vi "mupExpr Demo5.vi"() -> ()   [LabVIEW 2015]
uses:
  mupExpr/mupExpr.lvclass/mupExpr.ctl
  mupExpr/Set_SglVar_BulkMode_Value.vi
  mupExpr/Eval_BulkMode.vi
  mupExpr/Read Bulk Size.vi
  mupExpr/Read Expression.vi
  mupExpr/Read Singe Var Name.vi
  mupExpr/Read Variable_Names.vi
  mupLib/mupSetVarValue_Array.vi
  mupLib/mupEvalBulk.vi
  mupLib/mupCheckError.vi
  mupLib/mupLibPath.vi
  <vilib>/Utility/error.llb/Error Cluster From Error Code.vi
  mupExpr/mupExpr.lvclass
panel:
  in  "varValue":dbl[](array[numeric])=[0.0, 1.0, 2.0, 3.0, 4.0, 5.0]
  out "Result":dbl[](array[numeric]) format="%#_13g"
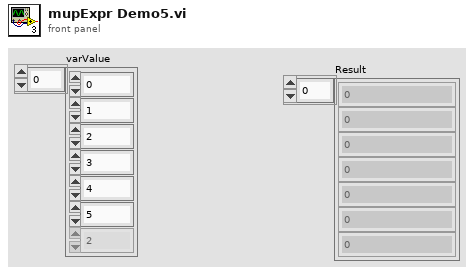
[diagram p1: front panel]
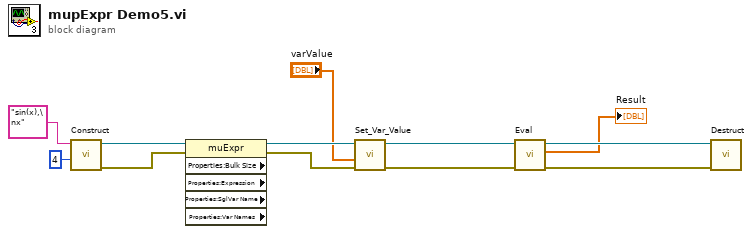
[diagram p0: block diagram]
diagram:
  n1 = call "Construct.vi"("Bulk Size (1)"=4, "Expression"="sin(x),\nx") -> ("error out"=w1:errorcluster, "mupExpr out"=w2:refnum<data-value>)  [unwired: 7 in, 1 out]
  n2 = property class="muExpr" props=["Properties:Bulk Size", "Properties:Expression", "Properties:SglVar Name", "Properties:Var Names"](reference=w2, error in=w1) -> (reference out=w7:refnum<data-value>, error out=w6:errorcluster)  [unwired: 4 out]
  n3 = call-poly "Set_Var_Value.vi"("error in (no error)"=w6, "varValue"="varValue", "mupExpr in"=w7) -> ("error out"=w10:errorcluster, "mupExpr out"=w11:refnum<data-value>)  [unwired: 7 in]
  n4 = call-poly "Eval.vi"("error in (no error)"=w10, "mupExpr in"=w11) -> ("error out"=w8:errorcluster, "Result"=→"Result":dbl[], "mupExpr out"=w9:refnum<data-value>)  [unwired: 7 in]
  n5 = call "Destruct.vi"("error in (no error)"=w8, "mupExpr in"=w9) -> ()  [unwired: 9 in, 1 out]
